vi "is_experiment_finished.vi"(8 "error in (no error)":errorcluster, 11 "DL090130ExperimentController in":refnum<class "ExperimentControllerDL090130Interval.lvclass">) -> (0 "error out":errorcluster, 2 "is finished?":bool, 3 "DL090130ExperimentController out":refnum<class "ExperimentControllerDL090130Interval.lvclass">)   [LabVIEW 2010, in "ExperimentControllerDL090130Interval.lvclass"]
uses:
  ExperimentControllerDL090130Interval.lvclass
  ExperimentControllerDL090130Interval.lvclass/ExperimentControllerDL090130Interval.ctl
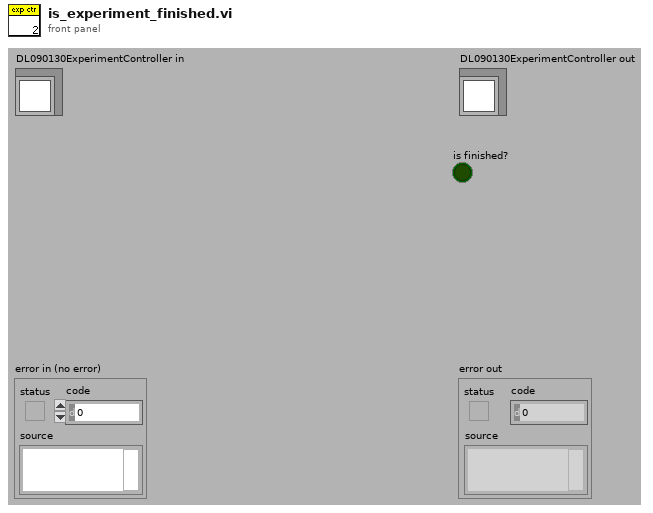
[diagram p1: front panel]
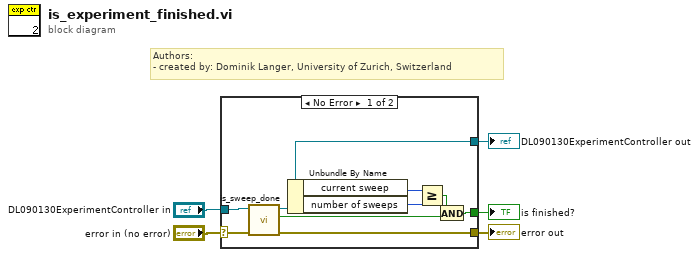
[diagram p0: block diagram]
diagram:
  # "Authors: \n- created by: Dominik Langer, University of Zurich, Switzerland"
  n1 = case shown="No Error" "error in (no error)" {
    selector: "error in (no error)" -> [w10 w16]
    tunnel: [w9 w16] -> w4
    tunnel: [w11 w15] -> w2
    tunnel: "DL090130ExperimentController in" -> [w12 w15]
    tunnel: [w6 _] -> w1
    frame No Error {
      n2 = call-dynamic "is_sweep_done.vi"("error in (no error)"=w10, "ExperimentControllerDL090130Interval in"=w12) -> ("error out"=w9:errorcluster, "sweep done?"=w8:bool, "ExperimentControllerDL090130Interval out"=w11:refnum<class "ExperimentControllerDL090130Interval.lvclass">)  [unwired: 7 in]
      n3 = Unbundle By Name(w11) -> ("current sweep"=w14:i32, "number of sweeps"=w13:i32)
      n4 = Greater Or Equal?(x=w14, y=w13) -> (x >= y?=w7:bool)
      n5 = And(x=w7, y=w8) -> (x .and. y?=w6:bool)
    }
    frame Error {
    }
  }
  "error out" <- w4
  "DL090130ExperimentController out" <- w2
  "is finished?" <- w1
